vi "InitDev.vi"(1 "SAVE?":bool, 2 "IP地址":string="192.168.1.16", 3 "SampleRate":T2(ring)=enum."105.468", 4 "SavePath":path) -> (0 "输出簇":T1)   [LabVIEW 2012]
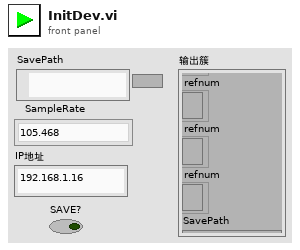
[diagram p1: front panel]
types:
  T1 = cluster{"refnum":refnum<file>, "refnum":refnum<file>, "refnum":refnum<file>, "refnum":refnum<file>, "refnum":refnum<file>, "SavePath":path, "SAVE?":bool, "connection ID":refnum<k5>}
  T2 = enum16{"", "105.468", "52.734", "35.156", "26.367", "21.094", "17.578", "15.067", "13.184", "11.719", "10.545"}
  T3 = enum16{"open", "replace", "create", "open or create", "replace or create", "replace or create with confirmation"}
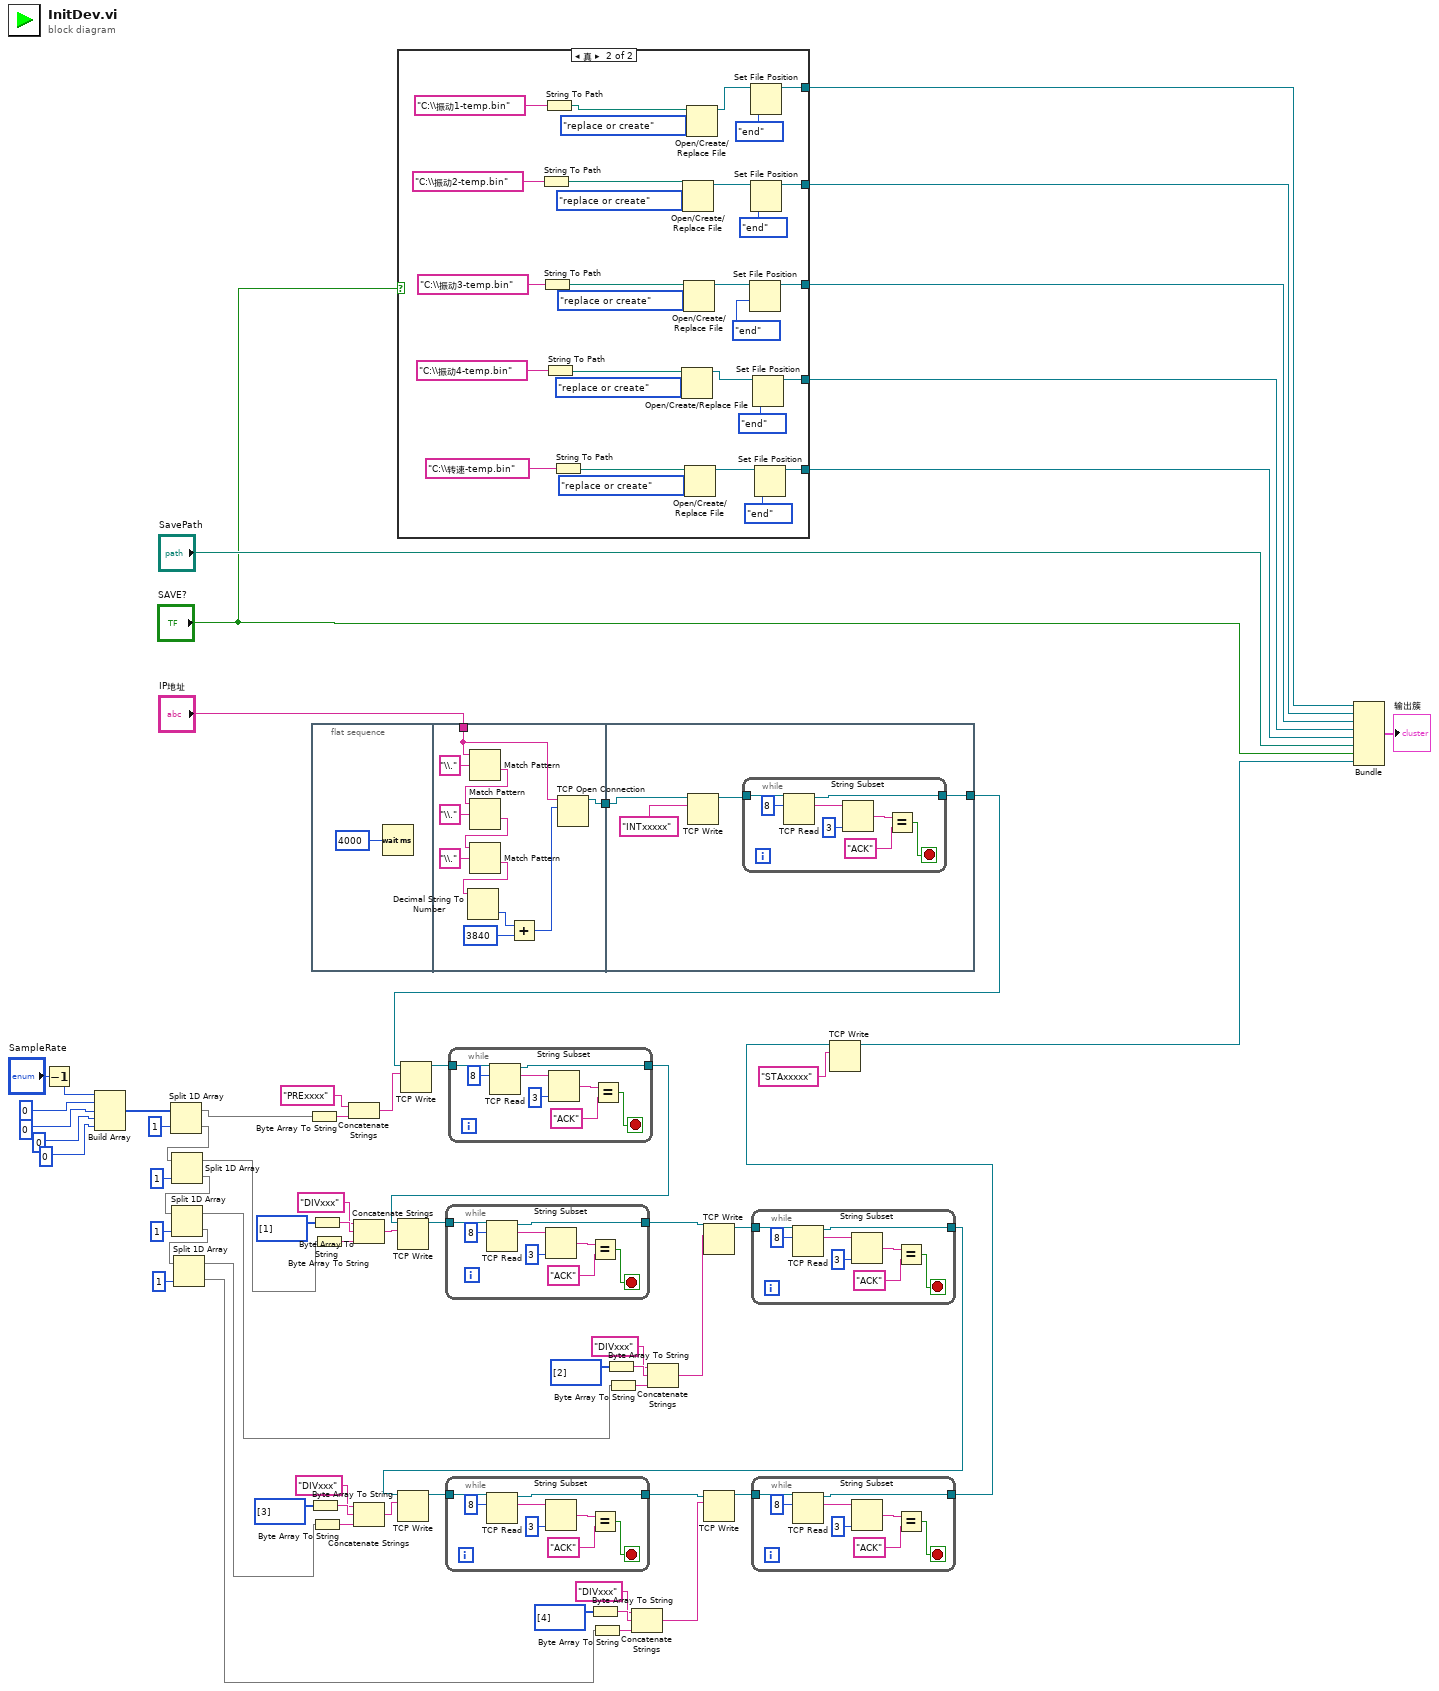
[diagram p0: block diagram]
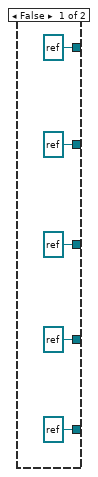
[diagram p2: hidden frame]
diagram:
  n1 = Decrement(x="SampleRate") -> (x-1=w8:T2)
  n2 = Build Array(w8, u8 0 ("元素"), u8 0 ("元素"), u8 0 ("元素"), u8 0 ("元素")) -> (w64:u16[])
  n3 = Split 1D Array(array=w64, index=1 ("索引")) -> (first subarray=w45:u16[], second subarray=w41:u16[])
  n4 = Split 1D Array(array=w41, index=1 ("索引")) -> (first subarray=w21:u16[], second subarray=w40:u16[])
  n5 = Split 1D Array(array=w40, index=1 ("索引")) -> (first subarray=w20:u16[], second subarray=w39:u16[])
  n6 = Split 1D Array(array=w39, index=1 ("索引")) -> (first subarray=w19:u16[], second subarray=w18:u16[])
  n7 = Byte Array To String(unsigned byte array=w45) -> (string=w49:string)
  n8 = Byte Array To String(unsigned byte array=u8[] [3] ("无符号字节数组")) -> (string=w27:string)
  n9 = flat-sequence {
    tunnel: [w77] -> w65
    tunnel: "IP地址" -> [w68]
    tunnel: w65 -> [w80]
    tunnel: [w78] -> w12
    frame #0 {
      n10 = Wait (ms)(milliseconds to wait=u32 4000 ("毫秒倍数")) -> ()  [unwired: 1 out]
    }
    frame #1 {
      n11 = Match Pattern(string=w68, regular expression="\\." ("正则表达式")) -> (after substring=w72:string)  [unwired: 1 in, 3 out]
      n12 = Match Pattern(string=w72, regular expression="\\." ("正则表达式")) -> (after substring=w73:string)  [unwired: 1 in, 3 out]
      n13 = Match Pattern(string=w73, regular expression="\\." ("正则表达式")) -> (after substring=w74:string)  [unwired: 1 in, 3 out]
      n14 = Decimal String To Number(string=w74) -> (number=w75:i32)  [unwired: 2 in, 1 out]
      n15 = Add(x=w75, y=3840) -> (x+y=w67:i32)
      n16 = TCP Open Connection(address=w68, remote port or service name=w67) -> (connection ID=w77:refnum<k5>)  [unwired: 3 in, 1 out]
    }
    frame #2 {
      n17 = TCP Write(connection ID=w80, data in="INTxxxxx" ("数据输入")) -> (connection ID out=w79:refnum<k5>)  [unwired: 2 in, 2 out]
      n18 = while {
        tunnel: w79 -> [w89]
        tunnel: [w83] -> w78
        stop <- w84 stop-if-true
        n19 = TCP Read(connection ID=w89, bytes to read=8 ("读取的字节")) -> (connection ID out=w83:refnum<k5>, data out=w87:string)  [unwired: 3 in, 1 out]
        n20 = String Subset(string=w87, length (rest)=3 ("偏移量(0)")) -> (substring=w86:string)  [unwired: 1 in]
        n21 = Equal?(x=w86, y="ACK") -> (x = y?=w84:bool)
      }
    }
  }
  n22 = Byte Array To String(unsigned byte array=u8[] [1] ("无符号字节数组")) -> (string=w35:string)
  n23 = Byte Array To String(unsigned byte array=w19) -> (string=w29:string)
  n24 = Byte Array To String(unsigned byte array=w21) -> (string=w38:string)
  n25 = Concatenate Strings("PRExxxx" ("数据输入"), w49) -> (w47:string)
  n26 = Concatenate Strings("DIVxxx" ("数据输入"), w35, w38) -> (w37:string)
  n27 = Concatenate Strings("DIVxxx" ("数据输入"), w27, w29) -> (w13:string)
  n28 = case shown="真" "SAVE?" {
    tunnel: [refnum<file> refnum ("refnum") w99] -> w7
    tunnel: [refnum<file> refnum ("refnum") w98] -> w6
    tunnel: [refnum<file> refnum ("refnum") w97] -> w5
    tunnel: [refnum<file> refnum ("refnum") w96] -> w4
    tunnel: [refnum<file> refnum ("refnum") w95] -> w3
    frame False {
    }
    frame True {
      n29 = String To Path(string="C:\\振动2-temp.bin" ("字符串")) -> (path=w113:path)
      n30 = String To Path(string="C:\\振动3-temp.bin" ("字符串")) -> (path=w112:path)
      n31 = String To Path(string="C:\\振动1-temp.bin" ("字符串")) -> (path=w114:path)
      n32 = String To Path(string="C:\\振动4-temp.bin" ("字符串")) -> (path=w111:path)
      n33 = String To Path(string="C:\\转速-temp.bin" ("字符串")) -> (path=w110:path)
      n34 = Open/Create/Replace File(file path (use dialog)=w111, operation (0:open)=T3."replace or create" ("操作(0:open)")) -> (refnum out=w121:refnum<file>)  [unwired: 4 in, 2 out]
      n35 = Open/Create/Replace File(file path (use dialog)=w113, operation (0:open)=T3."replace or create" ("操作(0:open)")) -> (refnum out=w123:refnum<file>)  [unwired: 4 in, 2 out]
      n36 = Open/Create/Replace File(file path (use dialog)=w112, operation (0:open)=T3."replace or create" ("操作(0:open)")) -> (refnum out=w122:refnum<file>)  [unwired: 4 in, 2 out]
      n37 = Open/Create/Replace File(file path (use dialog)=w110, operation (0:open)=T3."replace or create" ("操作(0:open)")) -> (refnum out=w120:refnum<file>)  [unwired: 4 in, 2 out]
      n38 = Open/Create/Replace File(file path (use dialog)=w114, operation (0:open)=T3."replace or create" ("操作(0:open)")) -> (refnum out=w124:refnum<file>)  [unwired: 4 in, 2 out]
      n39 = Set File Position(refnum=w122, from (0:start)=enum16{"start", "end", "current"}."end" ("自（0:起始）")) -> (refnum out=w97:refnum<file>)  [unwired: 2 in, 1 out]
      n40 = Set File Position(refnum=w124, from (0:start)=enum16{"start", "end", "current"}."end" ("自（0:起始）")) -> (refnum out=w99:refnum<file>)  [unwired: 2 in, 1 out]
      n41 = Set File Position(refnum=w123, from (0:start)=enum16{"start", "end", "current"}."end" ("自（0:起始）")) -> (refnum out=w98:refnum<file>)  [unwired: 2 in, 1 out]
      n42 = Set File Position(refnum=w121, from (0:start)=enum16{"start", "end", "current"}."end" ("自（0:起始）")) -> (refnum out=w96:refnum<file>)  [unwired: 2 in, 1 out]
      n43 = Set File Position(refnum=w120, from (0:start)=enum16{"start", "end", "current"}."end" ("自（0:起始）")) -> (refnum out=w95:refnum<file>)  [unwired: 2 in, 1 out]
    }
  }
  n44 = TCP Write(connection ID=w12, data in=w47) -> (connection ID out=w58:refnum<k5>)  [unwired: 2 in, 2 out]
  n45 = while {
    tunnel: w58 -> [w132]
    tunnel: [w126] -> w53
    stop <- w127 stop-if-true
    n46 = TCP Read(connection ID=w132, bytes to read=8 ("读取的字节")) -> (connection ID out=w126:refnum<k5>, data out=w130:string)  [unwired: 3 in, 1 out]
    n47 = String Subset(string=w130, length (rest)=3 ("偏移量(0)")) -> (substring=w129:string)  [unwired: 1 in]
    n48 = Equal?(x=w129, y="ACK") -> (x = y?=w127:bool)
  }
  n49 = TCP Write(connection ID=w53, data in=w37) -> (connection ID out=w57:refnum<k5>)  [unwired: 2 in, 2 out]
  n50 = while {
    tunnel: w57 -> [w140]
    tunnel: [w134] -> w52
    stop <- w135 stop-if-true
    n51 = TCP Read(connection ID=w140, bytes to read=8 ("读取的字节")) -> (connection ID out=w134:refnum<k5>, data out=w138:string)  [unwired: 3 in, 1 out]
    n52 = String Subset(string=w138, length (rest)=3 ("偏移量(0)")) -> (substring=w137:string)  [unwired: 1 in]
    n53 = Equal?(x=w137, y="ACK") -> (x = y?=w135:bool)
  }
  n54 = Byte Array To String(unsigned byte array=u8[] [4] ("无符号字节数组")) -> (string=w23:string)
  n55 = Byte Array To String(unsigned byte array=w18) -> (string=w25:string)
  n56 = Byte Array To String(unsigned byte array=u8[] [2] ("无符号字节数组")) -> (string=w31:string)
  n57 = Byte Array To String(unsigned byte array=w20) -> (string=w33:string)
  n58 = Concatenate Strings("DIVxxx" ("数据输入"), w23, w25) -> (w16:string)
  n59 = Concatenate Strings("DIVxxx" ("数据输入"), w31, w33) -> (w17:string)
  n60 = TCP Write(connection ID=w52, data in=w17) -> (connection ID out=w56:refnum<k5>)  [unwired: 2 in, 2 out]
  n61 = while {
    tunnel: w56 -> [w148]
    tunnel: [w142] -> w51
    stop <- w143 stop-if-true
    n62 = TCP Read(connection ID=w148, bytes to read=8 ("读取的字节")) -> (connection ID out=w142:refnum<k5>, data out=w146:string)  [unwired: 3 in, 1 out]
    n63 = String Subset(string=w146, length (rest)=3 ("偏移量(0)")) -> (substring=w145:string)  [unwired: 1 in]
    n64 = Equal?(x=w145, y="ACK") -> (x = y?=w143:bool)
  }
  n65 = TCP Write(connection ID=w51, data in=w13) -> (connection ID out=w55:refnum<k5>)  [unwired: 2 in, 2 out]
  n66 = while {
    tunnel: w55 -> [w156]
    tunnel: [w150] -> w50
    stop <- w151 stop-if-true
    n67 = TCP Read(connection ID=w156, bytes to read=8 ("读取的字节")) -> (connection ID out=w150:refnum<k5>, data out=w154:string)  [unwired: 3 in, 1 out]
    n68 = String Subset(string=w154, length (rest)=3 ("偏移量(0)")) -> (substring=w153:string)  [unwired: 1 in]
    n69 = Equal?(x=w153, y="ACK") -> (x = y?=w151:bool)
  }
  n70 = TCP Write(connection ID=w50, data in=w16) -> (connection ID out=w54:refnum<k5>)  [unwired: 2 in, 2 out]
  n71 = while {
    tunnel: w54 -> [w164]
    tunnel: [w158] -> w15
    stop <- w159 stop-if-true
    n72 = TCP Read(connection ID=w164, bytes to read=8 ("读取的字节")) -> (connection ID out=w158:refnum<k5>, data out=w162:string)  [unwired: 3 in, 1 out]
    n73 = String Subset(string=w162, length (rest)=3 ("偏移量(0)")) -> (substring=w161:string)  [unwired: 1 in]
    n74 = Equal?(x=w161, y="ACK") -> (x = y?=w159:bool)
  }
  n75 = TCP Write(connection ID=w15, data in="STAxxxxx" ("数据输入")) -> (connection ID out=w11:refnum<k5>)  [unwired: 2 in, 2 out]
  n76 = Bundle("refnum"=w7, "refnum"=w6, "refnum"=w5, "refnum"=w4, "refnum"=w3, "SavePath"="SavePath", "SAVE?"="SAVE?", "connection ID"=w11) -> (→"输出簇":T1)  [unwired: 1 in]
